vi "Hierarchy to Name.vi"(7 "Delimiter":string, 11 "Hierarchy":string[](array[string])) -> (3 "Full Name":string)   [LabVIEW 2020, in "CDM-Config.lvlib"]
doc: "Helper VI for concatenating hierarchy name elements into a single string using the specified delimiter."
uses:
  CDM-Config.lvlib
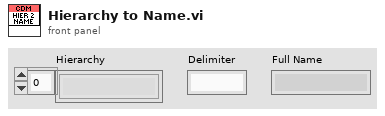
[diagram p1: front panel]
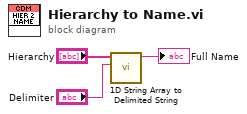
[diagram p0: block diagram]
diagram:
  n1 = call <vilib>:"1D String Array to Delimited String.vi"("delimiter"="Delimiter", "string array"="Hierarchy") -> ("delimited string"=→"Full Name":string)  [unwired: 9 in]
